vi "rs3_WriteDepthPreference3.vi"(1 "ST Color Control 2":T5, 2 "ST SLO Threshold 2":T3={"SLOdiffThreshRed(76)"=200, "SLODiffThreshGreen(77)"=200, "SLODiffThreshBlue(78)"=200}, 4 "ST_AE_Control":cluster{"meanIntensitySetpoint":u32}={"meanIntensitySetpoint"=800}, 5 "depth control 2":T9={"plusIncrement (47)"=19, "MinusDecrement (46)"=4, "deepSeaMedianThreshold (48)"=554, "scoreThreshA(49)"=1, "scoreThreshB (50)"=632, "textureDifferenceThreshold (52)"=0, "textureCountThreshold (51)"=32, "deepSea2ndPeakThresh.(53)"=665, "deepSeaNeighborThresh.(54)"=126, "IrAgreeThreshold (55)"=11}, 6 "Depth Table":T1={"depthUnits, um"=1000, "depthClampMin"=0, "depthClampMax"=65535, "disparityMultiplier"=0, "disparityShift(0-127)"=0}, 7 "ST RSM 2":T8={"rsmBypass (56)"=0, "diffThresh (57)"=6.49, "sloRauDiffThresh(58)"=0.305, "removeThresh(59)"=60}, 8 "ST_CensusEnable":cluster{"uDiameter":u32, "vDiameter":u32}={"uDiameter"=9, "vDiameter"=9}, 9 "ST SLO Penalty 2":T7={"sloK1Penalty (79)"=10, "sloK2Penalty (80)"=60, "sloK1PenaltyMod1(81)"=84, "sloK2PenaltyMod1(82)"=56, "sloK1PenaltyMod2(83)"=59, "sloK2PenaltyMod2(84)"=4}, 11 "ST RAU vector 2":T6={"minWest (60)"=7, "minEast (61)"=7, "minWEsum (62)"=12, "minNorth (63)"=3, "minSouth (64)"=2, "minNSSum(65)"=1, "uStrink (66)"=2, "vShrink (67)"=1}, 12 "ST Rau Threshold 2":T4={"rauDiffThreshRed(73)"=70, "rauDiffThreshGreen(74)"=70, "rauDiffThreshBlue(75)"=70}, 13 "HDAD 2*":T2={"lambdaCensus"=126.0, "lambdaAD"=800.0, "ignoreSAD"=0}, 14 "error in (no error)":errorcluster) -> (15 "error out":errorcluster={"status"=TRUE, "code"=1430, "source"="Write to Text File in RS2_WriteDepthPreference2.vi<APPEND>\n"})   [LabVIEW 2017, in "libRealSense3.lvlib"]
uses:
  libRealSense3.lvlib
panel:
  out "NewJSON":string
  # "RS2 Write Depth Preferences 3"
  # "{\n    \"param-censususize\": 9,\n    \"param-censusvsize\": 9,\n    \"param-disableraucolor\": 0,\n    \"param-disablesadcolor\": 0,\n    \"param-disablesadnormalize\": 0,\n    \"param-disablesloleftcolor\": 0,\n    \"param-disableslorightcolor\": 0,\n    \"param-lambdaad\": 800,\n    \"param-lambdacensus\": 26,\n    \"param-leftrightthreshold\": 24,\n    \"param-maxscorethreshb\": 2047,\n    \"param-medianthreshold\": 500,\n    \"param-minscorethresha\": 1,\n    \"param-neighborthresh\": 7,\n    \"param-raumine\": 1,\n    \"param-rauminn\": 1,\n    \"param-rauminnssum\": 3,\n    \"param-raumins\": 1,\n    \"param-rauminw\": 1,\n    \"param-rauminwesum\": 3,\n    \"param-regioncolorthresholdb\": 0.05,\n    \"param-regioncolorthresholdg\": 0.05,\n    \"param-regioncolorthresholdr\": 0.05,\n    \"param-regionshrinku\": 3,\n    \"param-regionshrinkv\": 1,\n    \"param-regionspatialthresholdu\": 7,\n    \"param-regionspatialthresholdv\": 3,\n    \"param-robbinsmonrodecrement\": 10,\n    \"param-robbinsmonroincrement\": 10,\n    \"param-rsmdiffthreshold\": 4.0,\n    \"param-rsmrauslodiffthreshold\": 1.0,\n    \"param-rsmremovethreshold\": 0.3,\n    \"param-scanlineedgetaub\": 72,\n    \"param-scanlineedgetaug\": 72,\n    \"param-scanlineedgetaur\": 72,\n    \"param-scanlinep1\": 180,\n    \"param-scanlinep1onediscon\": 90,\n    \"param-scanlinep1twodiscon\": 59,\n    \"param-scanlinep2\": 342,\n    \"param-scanlinep2onediscon\": 171,\n    \"param-scanlinep2twodiscon\": 113,\n    \"param-secondpeakdelta\": 675,\n    \"param-texturecountthresh\": 0,\n    \"param-texturedifferencethresh\": 0,\n    \"param-usersm\": 1\n}"
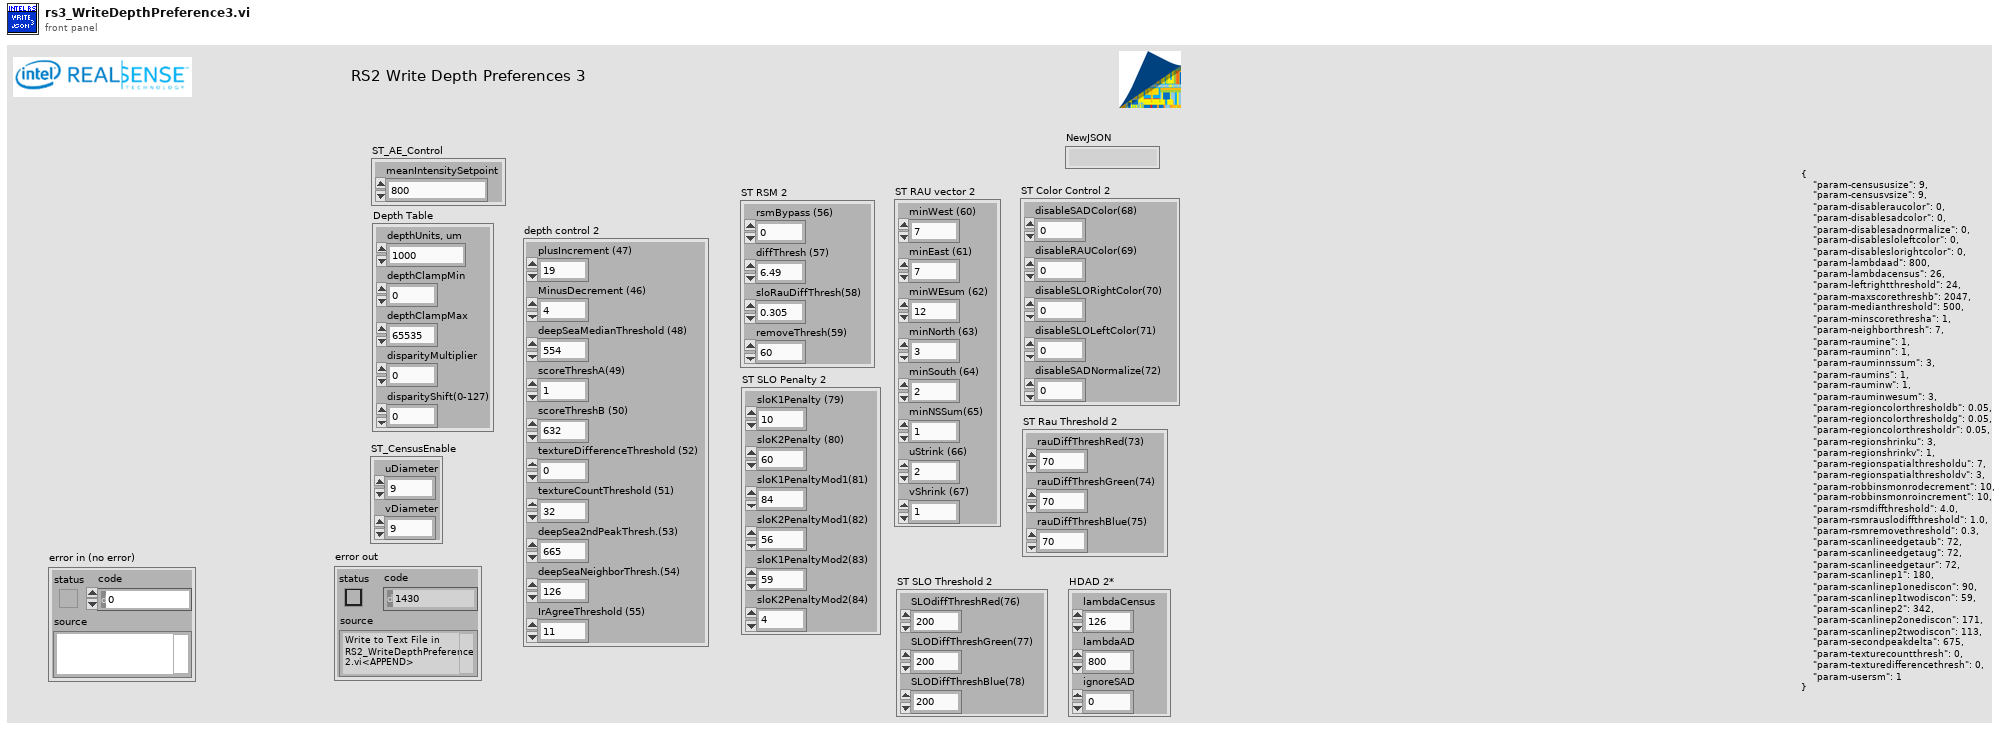
[diagram p1: front panel]
types:
  T1 = cluster{"depthUnits, um":u32, "depthClampMin":u32, "depthClampMax":u32, "disparityMultiplier":u32, "disparityShift(0-127)":u32}
  T2 = cluster{"lambdaCensus":sgl, "lambdaAD":sgl, "ignoreSAD":u32}
  T3 = cluster{"SLOdiffThreshRed(76)":u32, "SLODiffThreshGreen(77)":u32, "SLODiffThreshBlue(78)":u32}
  T4 = cluster{"rauDiffThreshRed(73)":u32, "rauDiffThreshGreen(74)":u32, "rauDiffThreshBlue(75)":u32}
  T5 = cluster{"disableSADColor(68)":u32, "disableRAUColor(69)":u32, "disableSLORightColor(70)":u32, "disableSLOLeftColor(71)":u32, "disableSADNormalize(72)":u32}
  T6 = cluster{"minWest (60)":u32, "minEast (61)":u32, "minWEsum (62)":u32, "minNorth (63)":u32, "minSouth (64)":u32, "minNSSum(65)":u32, "uStrink (66)":u32, "vShrink (67)":u32}
  T7 = cluster{"sloK1Penalty (79)":u32, "sloK2Penalty (80)":u32, "sloK1PenaltyMod1(81)":u32, "sloK2PenaltyMod1(82)":u32, "sloK1PenaltyMod2(83)":u32, "sloK2PenaltyMod2(84)":u32}
  T8 = cluster{"rsmBypass (56)":u32, "diffThresh (57)":sgl, "sloRauDiffThresh(58)":sgl, "removeThresh(59)":u32}
  T9 = cluster{"plusIncrement (47)":u32, "MinusDecrement (46)":u32, "deepSeaMedianThreshold (48)":u32, "scoreThreshA(49)":u32, "scoreThreshB (50)":u32, "textureDifferenceThreshold (52)":u32, "textureCountThreshold (51)":u32, "deepSea2ndPeakThresh.(53)":u32, "deepSeaNeighborThresh.(54)":u32, "IrAgreeThreshold (55)":u32}
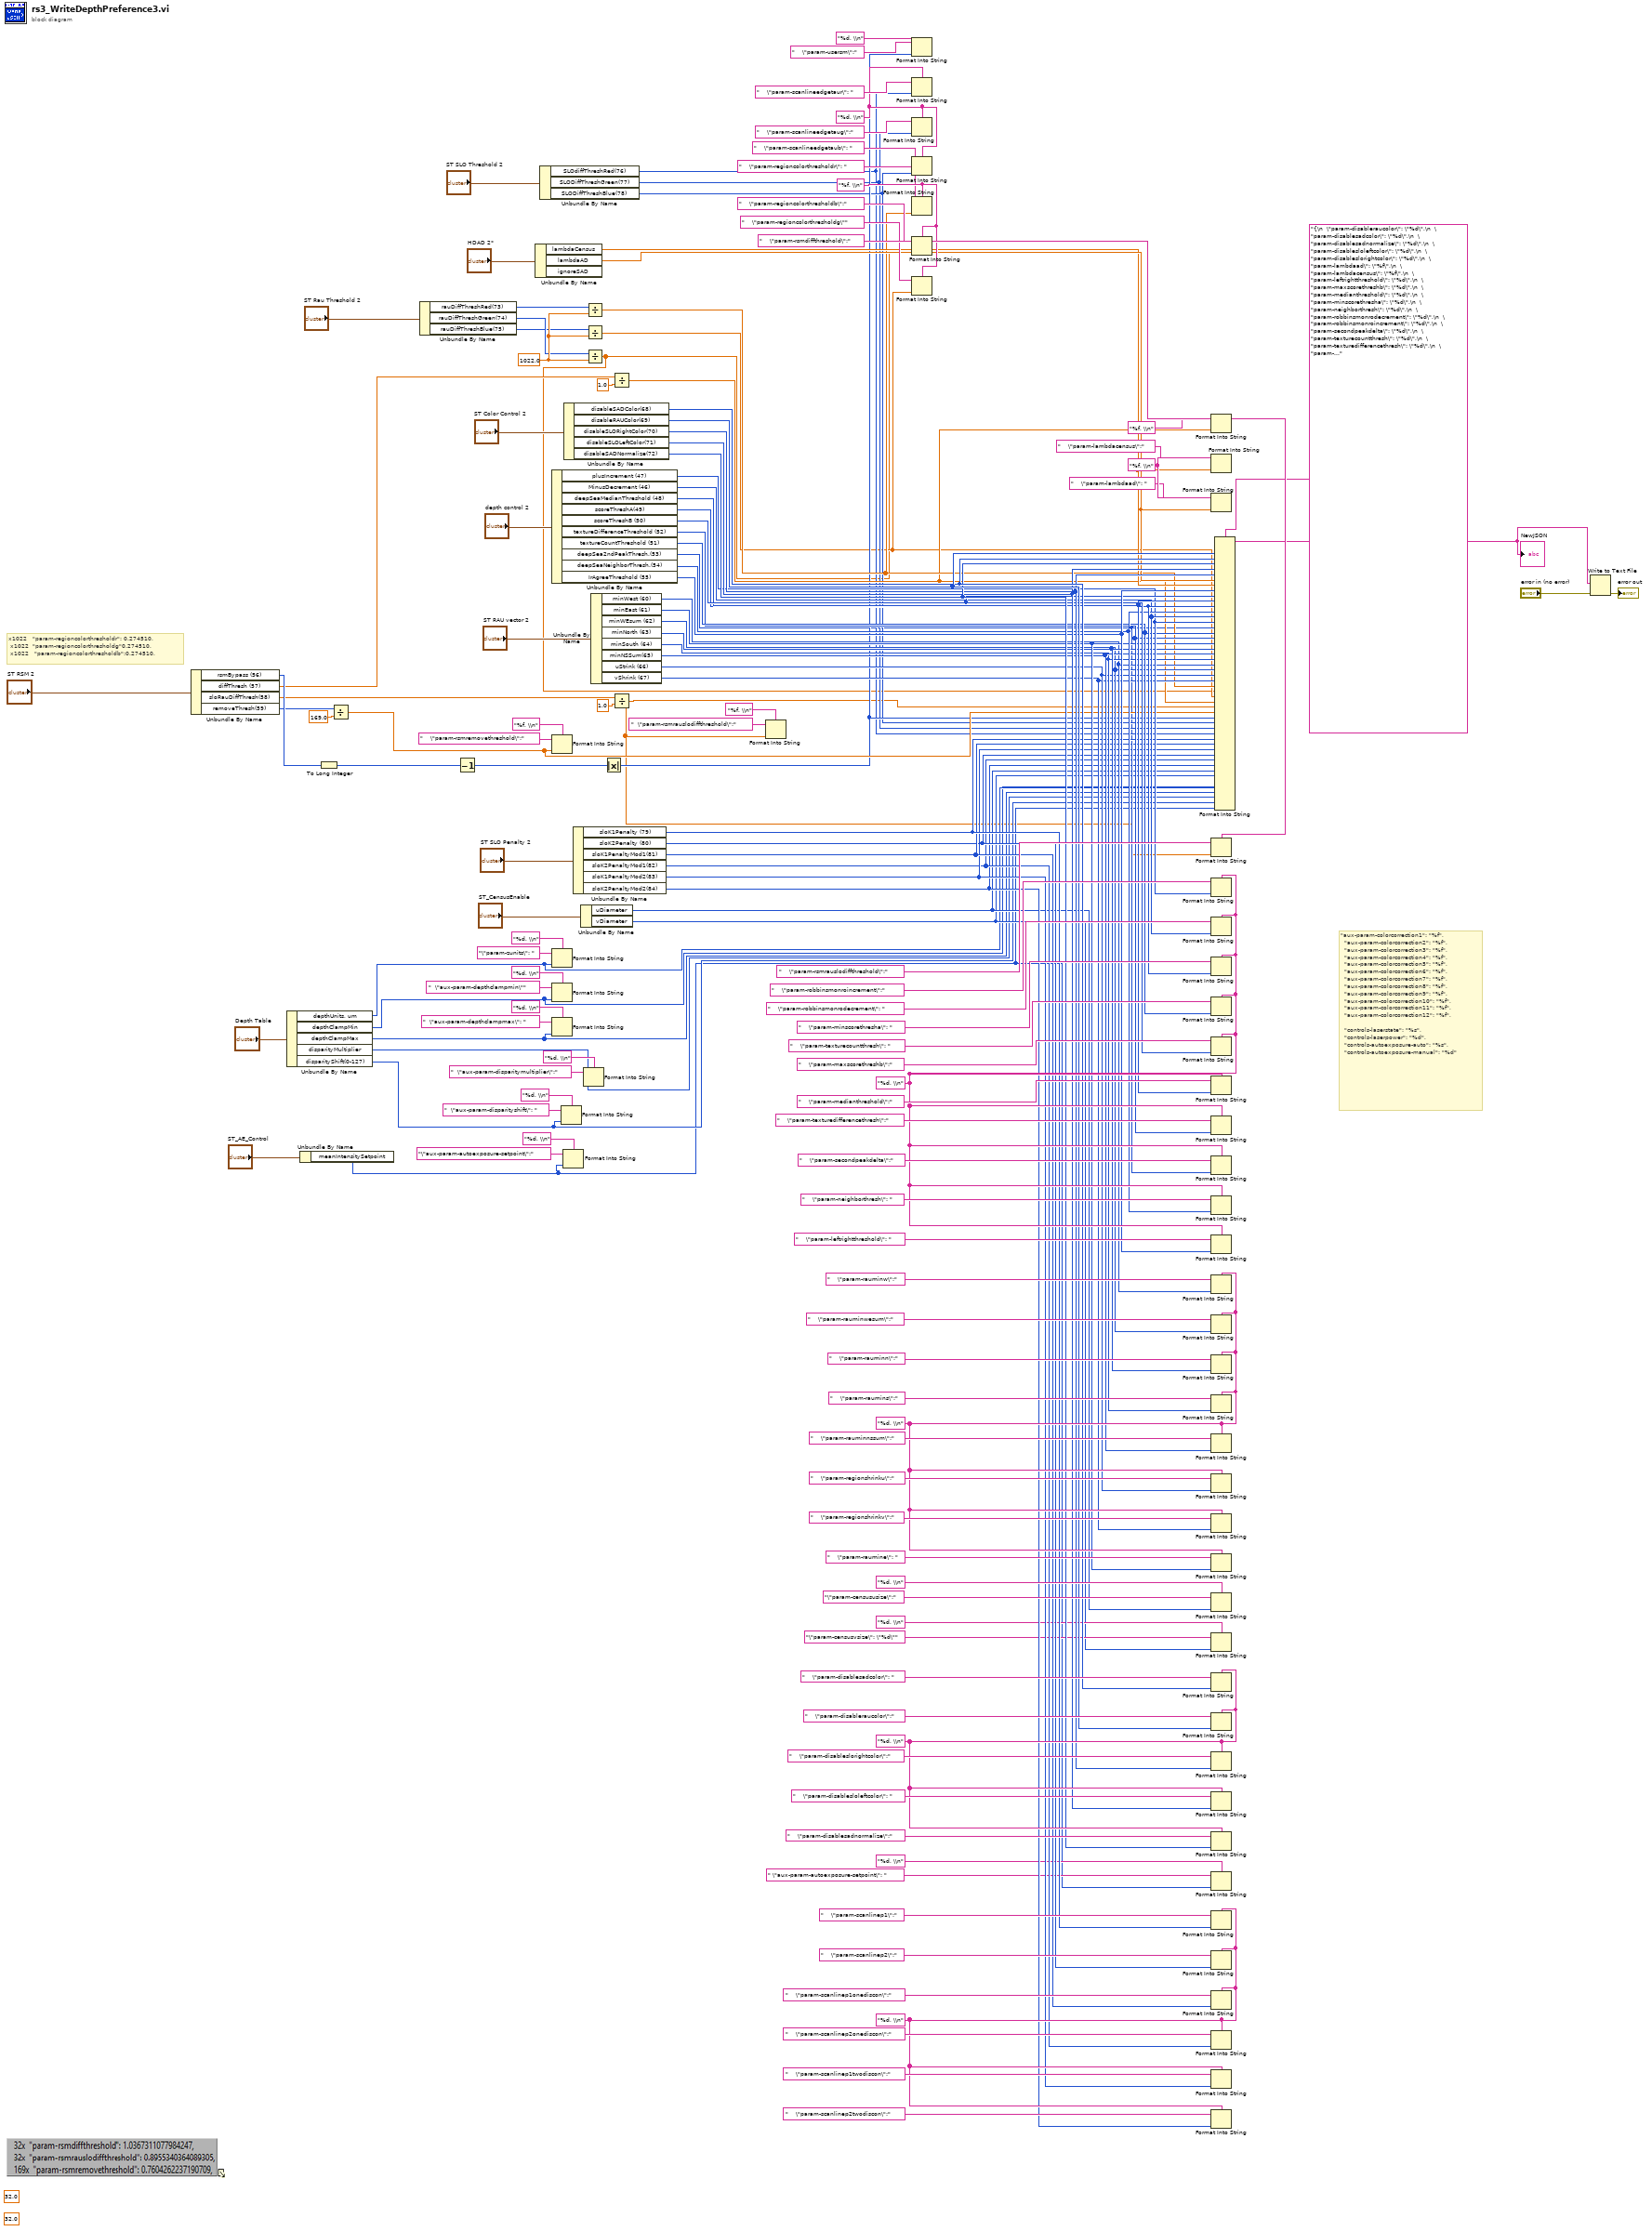
[diagram p0: block diagram]
diagram:
  (unwired) 32.0 ("x")
  (unwired) 32.0 ("x")
  w82 = 1022.0 ("y")
  w95 = "%f, \\n" ("format string")
  w86 = "%d, \\n" ("format string")
  w97 = "%f, \\n" ("format string")
  w101 = "%d, \\n" ("format string")
  w108 = "%d, \\n" ("format string")
  w118 = "%d, \\n" ("format string")
  w130 = "%f, \\n" ("format string")
  w137 = "%d, \\n" ("format string")
  # "\"aux-param-colorcorrection1\": \"%f\",\n  \"aux-param-colorcorrection2\": \"%f\",\n  \"aux-param-colorcorrection3\": \"%f\",\n  \"aux-param-colorcorrection4\": \"%f\",\n  \"aux-param-colorcorrection5\": \"%f\",\n  \"aux-param-colorcorrection6\": \"%f\",\n  \"aux-param-colorcorrection7\": \"%f\",\n  \"aux-param-colorcorrection8\": \"%f\",\n  \"aux-param-colorcorrection9\": \"%f\",\n  \"aux-param-colorcorrection10\": \"%f\",\n  \"aux-param-colorcorrection11\": \"%f\",\n  \"aux-param-colorcorrection12\": \"%f\",\n\n  \"controls-laserstate\": \"%s\",\n  \"controls-laserpower\": \"%d\",\n  \"controls-autoexposure-auto\": \"%s\",\n  \"controls-autoexposure-manual\": \"%d\""
  # "x1022   \"param-regioncolorthresholdr\": 0.274510, \n x1022  \"param-regioncolorthresholdg\"0.274510, \n x1022   \"param-regioncolorthresholdb\":0.274510,"
  n1 = Unbundle By Name("ST RSM 2") -> ("rsmBypass (56)"=w129:u32, "diffThresh (57)"=w76:sgl, "sloRauDiffThresh(58)"=w73:sgl, "removeThresh(59)"=w74:u32)
  n2 = Unbundle By Name("Depth Table") -> ("depthUnits, um"=w16:u32, "depthClampMin"=w15:u32, "depthClampMax"=w14:u32, "disparityMultiplier"=w13:u32, "disparityShift(0-127)"=w12:u32)
  n3 = Unbundle By Name("ST_AE_Control") -> ("meanIntensitySetpoint"=w6:u32)
  n4 = To Long Integer(number=w129) -> (32bit integer=w127:i32)
  n5 = Divide(x=w74, y=169.0 ("x")) -> (x/y=w45:dbl)
  n6 = Unbundle By Name("ST Rau Threshold 2") -> ("rauDiffThreshRed(73)"=w81:u32, "rauDiffThreshGreen(74)"=w80:u32, "rauDiffThreshBlue(75)"=w79:u32)
  n7 = Decrement(x=w127) -> (x-1=w128:i32)
  n8 = Unbundle By Name("HDAD 2*") -> ("lambdaCensus"=w65:sgl, "lambdaAD"=w66:sgl)  [unwired: 1 out]
  n9 = Unbundle By Name("ST SLO Threshold 2") -> ("SLOdiffThreshRed(76)"=w41:u32, "SLODiffThreshGreen(77)"=w42:u32, "SLODiffThreshBlue(78)"=w43:u32)
  n10 = Unbundle By Name("depth control 2") -> ("plusIncrement (47)"=w58:u32, "MinusDecrement (46)"=w59:u32, "deepSeaMedianThreshold (48)"=w62:u32, "scoreThreshA(49)"=w61:u32, "scoreThreshB (50)"=w63:u32, "textureDifferenceThreshold (52)"=w56:u32, "textureCountThreshold (51)"=w57:u32, "deepSea2ndPeakThresh.(53)"=w39:u32, "deepSeaNeighborThresh.(54)"=w60:u32, "IrAgreeThreshold (55)"=w64:u32)
  n11 = Format Into String(format string="%f, \\n", initial string="    \"param-rsmremovethreshold\":" ("regular expression"), w45) -> ()  [unwired: 1 in, 2 out]
  n12 = Format Into String(format string="%d, \\n", initial string="\"param-zunits\": " ("regular expression"), w16) -> ()  [unwired: 1 in, 2 out]
  n13 = Format Into String(format string="%d, \\n", initial string="  \"aux-param-depthclampmin\"" ("regular expression"), w15) -> ()  [unwired: 1 in, 2 out]
  n14 = Format Into String(format string="%d, \\n", initial string="  \"aux-param-depthclampmax\": " ("regular expression"), w14) -> ()  [unwired: 1 in, 2 out]
  n15 = Format Into String(format string="%d, \\n", initial string="  \"aux-param-disparityshift\": " ("regular expression"), w12) -> ()  [unwired: 1 in, 2 out]
  n16 = Format Into String(format string="%d, \\n", initial string="\"aux-param-autoexposure-setpoint\":" ("regular expression"), w6) -> ()  [unwired: 1 in, 2 out]
  n17 = Unbundle By Name("ST Color Control 2") -> ("disableSADColor(68)"=w71:u32, "disableRAUColor(69)"=w72:u32, "disableSLORightColor(70)"=w68:u32, "disableSLOLeftColor(71)"=w69:u32, "disableSADNormalize(72)"=w70:u32)
  n18 = Unbundle By Name("ST SLO Penalty 2") -> ("sloK1Penalty (79)"=w40:u32, "sloK2Penalty (80)"=w35:u32, "sloK1PenaltyMod1(81)"=w37:u32, "sloK2PenaltyMod1(82)"=w34:u32, "sloK1PenaltyMod2(83)"=w36:u32, "sloK2PenaltyMod2(84)"=w33:u32)
  n19 = Unbundle By Name("ST_CensusEnable") -> ("uDiameter"=w29:u32, "vDiameter"=w28:u32)
  n20 = Format Into String(format string="%d, \\n", initial string="  \"aux-param-disparitymultiplier\":" ("regular expression"), w13) -> ()  [unwired: 1 in, 2 out]
  n21 = Divide(x=w81, y=w82) -> (x/y=w47:dbl)
  n22 = Divide(x=w79, y=w82) -> (x/y=w2:dbl)
  n23 = Divide(x=w80, y=w82) -> (x/y=w1:dbl)
  n24 = Unbundle By Name("ST RAU vector 2") -> ("minWest (60)"=w51:u32, "minEast (61)"=w55:u32, "minWEsum (62)"=w50:u32, "minNorth (63)"=w54:u32, "minSouth (64)"=w52:u32, "minNSSum(65)"=w53:u32, "uStrink (66)"=w49:u32, "vShrink (67)"=w48:u32)
  n25 = Absolute Value(x=w128) -> (abs(x)=w44:i32)
  n26 = Divide(x=w76, y=1.0 ("x")) -> (x/y=w46:dbl)
  n27 = Divide(x=w73, y=1.0 ("x")) -> (x/y=w3:dbl)
  n28 = Format Into String(format string="%f, \\n", initial string="  \"param-rsmrauslodiffthreshold\":" ("regular expression"), w3) -> ()  [unwired: 1 in, 2 out]
  n29 = Format Into String(format string="%d, \\n", initial string="    \"param-usersm\":" ("regular expression"), w44) -> ()  [unwired: 1 in, 2 out]
  n30 = Format Into String(format string=w86, initial string="    \"param-scanlineedgetaur\": " ("regular expression"), w41) -> ()  [unwired: 1 in, 2 out]
  n31 = Format Into String(format string=w86, initial string="    \"param-scanlineedgetaug\":" ("regular expression"), w42) -> ()  [unwired: 1 in, 2 out]
  n32 = Format Into String(format string=w86, initial string="    \"param-scanlineedgetaub\": " ("regular expression"), w43) -> ()  [unwired: 1 in, 2 out]
  n33 = Format Into String(format string=w97, initial string="    \"param-regioncolorthresholdr\": " ("regular expression"), w47) -> ()  [unwired: 1 in, 2 out]
  n34 = Format Into String(format string=w97, initial string="    \"param-regioncolorthresholdb\":" ("regular expression"), w1) -> ()  [unwired: 1 in, 2 out]
  n35 = Format Into String(format string=w97, initial string="    \"param-regioncolorthresholdg\"" ("regular expression"), w2) -> ()  [unwired: 1 in, 2 out]
  n36 = Format Into String(format string=w130, initial string="    \"param-rsmdiffthreshold\":" ("regular expression"), w46) -> ()  [unwired: 1 in, 2 out]
  n37 = Format Into String(format string=w95, initial string="    \"param-lambdacensus\":" ("regular expression"), w65) -> ()  [unwired: 1 in, 2 out]
  n38 = Format Into String(format string=w95, initial string="    \"param-lambdaad\": " ("regular expression"), w66) -> ()  [unwired: 1 in, 2 out]
  n39 = Format Into String(format string=w130, initial string="    \"param-rsmrauslodiffthreshold\":" ("regular expression"), w3) -> ()  [unwired: 1 in, 2 out]
  n40 = Format Into String(format string=w137, initial string="    \"param-robbinsmonroincrement\":" ("regular expression"), w58) -> ()  [unwired: 1 in, 2 out]
  n41 = Format Into String(format string=w137, initial string="    \"param-robbinsmonrodecrement\": " ("regular expression"), w59) -> ()  [unwired: 1 in, 2 out]
  n42 = Format Into String(format string=w137, initial string="    \"param-minscorethresha\": " ("regular expression"), w61) -> ()  [unwired: 1 in, 2 out]
  n43 = Format Into String(format string=w137, initial string="    \"param-texturecountthresh\": " ("regular expression"), w57) -> ()  [unwired: 1 in, 2 out]
  n44 = Format Into String(format string=w137, initial string="    \"param-maxscorethreshb\":" ("regular expression"), w63) -> ()  [unwired: 1 in, 2 out]
  n45 = Format Into String(format string=w137, initial string="    \"param-medianthreshold\":" ("regular expression"), w62) -> ()  [unwired: 1 in, 2 out]
  n46 = Format Into String(format string=w137, initial string="    \"param-texturedifferencethresh\":" ("regular expression"), w56) -> ()  [unwired: 1 in, 2 out]
  n47 = Format Into String(format string=w137, initial string="    \"param-secondpeakdelta\":" ("regular expression"), w39) -> ()  [unwired: 1 in, 2 out]
  n48 = Format Into String(format string=w137, initial string="    \"param-neighborthresh\": " ("regular expression"), w60) -> ()  [unwired: 1 in, 2 out]
  n49 = Format Into String(format string=w137, initial string="    \"param-leftrightthreshold\": " ("regular expression"), w64) -> ()  [unwired: 1 in, 2 out]
  n50 = Format Into String(format string=w108, initial string="    \"param-rauminw\":" ("regular expression"), w51) -> ()  [unwired: 1 in, 2 out]
  n51 = Format Into String(format string=w108, initial string="    \"param-rauminwesum\":" ("regular expression"), w50) -> ()  [unwired: 1 in, 2 out]
  n52 = Format Into String(format string=w108, initial string="    \"param-rauminn\":" ("regular expression"), w54) -> ()  [unwired: 1 in, 2 out]
  n53 = Format Into String(format string=w108, initial string="    \"param-raumins\":" ("regular expression"), w52) -> ()  [unwired: 1 in, 2 out]
  n54 = Format Into String(format string=w108, initial string="    \"param-rauminnssum\":" ("regular expression"), w53) -> ()  [unwired: 1 in, 2 out]
  n55 = Format Into String(format string=w108, initial string="    \"param-regionshrinku\":" ("regular expression"), w49) -> ()  [unwired: 1 in, 2 out]
  n56 = Format Into String(format string=w108, initial string="    \"param-regionshrinkv\":" ("regular expression"), w48) -> ()  [unwired: 1 in, 2 out]
  n57 = Format Into String(format string=w108, initial string="    \"param-raumine\": " ("regular expression"), w55) -> ()  [unwired: 1 in, 2 out]
  n58 = Format Into String(format string="%d, \\n", initial string="\"param-censususize\":" ("regular expression"), w29) -> ()  [unwired: 1 in, 2 out]
  n59 = Format Into String(format string="%d, \\n", initial string="\"param-censusvsize\": \"%d\"" ("regular expression"), w28) -> ()  [unwired: 1 in, 2 out]
  n60 = Format Into String(format string=w101, initial string="    \"param-disablesadcolor\": " ("regular expression"), w71) -> ()  [unwired: 1 in, 2 out]
  n61 = Format Into String(format string=w101, initial string="    \"param-disableraucolor\":" ("regular expression"), w72) -> ()  [unwired: 1 in, 2 out]
  n62 = Format Into String(format string=w101, initial string="    \"param-disableslorightcolor\":" ("regular expression"), w68) -> ()  [unwired: 1 in, 2 out]
  n63 = Format Into String(format string=w101, initial string="    \"param-disablesloleftcolor\": " ("regular expression"), w69) -> ()  [unwired: 1 in, 2 out]
  n64 = Format Into String(format string=w101, initial string="    \"param-disablesadnormalize\":" ("regular expression"), w70) -> ()  [unwired: 1 in, 2 out]
  n65 = Format Into String(format string="%d, \\n", initial string=" \"aux-param-autoexposure-setpoint\": " ("regular expression"), w6) -> ()  [unwired: 1 in, 2 out]
  n66 = Format Into String(format string=w118, initial string="    \"param-scanlinep1\":" ("regular expression"), w40) -> ()  [unwired: 1 in, 2 out]
  n67 = Format Into String(format string=w118, initial string="    \"param-scanlinep2\":" ("regular expression"), w35) -> ()  [unwired: 1 in, 2 out]
  n68 = Format Into String(format string=w118, initial string="    \"param-scanlinep1onediscon\":" ("regular expression"), w37) -> ()  [unwired: 1 in, 2 out]
  n69 = Format Into String(format string=w118, initial string="    \"param-scanlinep2onediscon\":" ("regular expression"), w34) -> ()  [unwired: 1 in, 2 out]
  n70 = Format Into String(format string=w118, initial string="    \"param-scanlinep1twodiscon\":" ("regular expression"), w36) -> ()  [unwired: 1 in, 2 out]
  n71 = Format Into String(format string=w118, initial string="    \"param-scanlinep2twodiscon\":" ("regular expression"), w33) -> ()  [unwired: 1 in, 2 out]
  n72 = Format Into String(format string="{\n  \"param-disableraucolor\": \"%d\",\n  \"param-disablesadcolor\": \"%d\",\n  \"param-disablesadnormalize\": \"%d\",\n  \"param-disablesloleftcolor\": \"%d\",\n  \"param-disableslorightcolor\": \"%d\",\n  \"param-lambdaad\": \"%f\",\n  \"param-lambdacensus\": \"%f\",\n  \"param-leftrightthreshold\": \"%d\",\n  \"param-maxscorethreshb\": \"%d\",\n  \"param-medianthreshold\": \"%d\",\n  \"param-minscorethresha\": \"%d\",\n  \"param-neighborthresh\": \"%d\",\n  \"param-robbinsmonrodecrement\": \"%d\",\n  \"param-robbinsmonroincrement\": \"%d\",\n  \"param-secondpeakdelta\": \"%d\",\n  \"param-texturecountthresh\": \"%d\",\n  \"param-texturedifferencethresh\": \"%d\",\n  \"param-raumine\": \"%d\",\n  \"param-rauminn\": \"%d\",\n  \"param-rauminnssum\": \"%d\",\n  \"param-raumins\": \"%d\",\n  \"param-rauminw\": \"%d\",\n  \"param-rauminwesum\": \"%d\",\n  \"param-regionshrinku\": \"%d\",\n  \"param-regionshrinkv\": \"%d\",\n  \"param-regioncolorthresholdr\": \"%f\",\n  \"param-regioncolorthresholdg\": \"%f\",\n  \"param-regioncolorthresholdb\": \"%f\",\n  \"param-rsmdiffthreshold\": \"%f\",\n  \"param-rsmrauslodiffthreshold\": \"%f\",\n  \"param-rsmremovethreshold\": \"%f\",\n  \"param-usersm\": \"%d\",\n  \"param-scanlineedgetaub\": \"%d\",\n  \"param-scanlineedgetaug\": \"%d\",\n  \"param-scanlineedgetaur\": \"%d\",\n  \"param-scanlinep1\": \"%d\",\n  \"param-scanlinep1onediscon\": \"%d\",\n  \"param-scanlinep1twodiscon\": \"%d\",\n  \"param-scanlinep2\": \"%d\",\n  \"param-scanlinep2onediscon\": \"%d\",\n  \"param-scanlinep2twodiscon\": \"%d\",\n  \"param-censususize\": \"%d\",\n  \"param-censusvsize\": \"%d\",\n  \"param-zunits\": \"%d\",\n  \"aux-param-depthclampmin\": \"%d\",\n  \"aux-param-depthclampmax\": \"%d\",\n  \"aux-param-disparitymultiplier\": \"%d\",\n  \"aux-param-disparityshift\": \"%d\",\n  \"aux-param-autoexposure-setpoint\": \"%d\"\n}" ("regular expression"), w72, w71, w70, w69, w68, w66, w65, w64, w63, w62, w61, w60, w59, w58, w39, w57, w56, w55, w54, w53, w52, w51, w50, w49, w48, w47, w1, w2, w46, w3, w45, w44, w43, w42, w41, w40, w37, w36, w35, w34, w33, w29, w28, w16, w15, w14, w13, w12, w6) -> (resulting string=w38:string)  [unwired: 2 in, 1 out]
  "NewJSON" <- w38
  n73 = Write to Text File(text=w38, error in="error in (no error)") -> (error out=→"error out":errorcluster)  [unwired: 2 in, 2 out]
